vi "Que_Creat.vi"(8 "error in (no error)":errorcluster caption="error in", 11 "QueueName":string) -> (0 "error out":errorcluster, 3 "QueueName out":string)   [LabVIEW 2016]
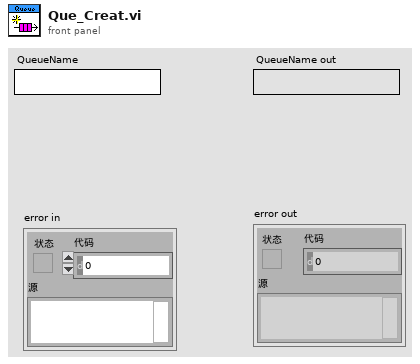
[diagram p1: front panel]
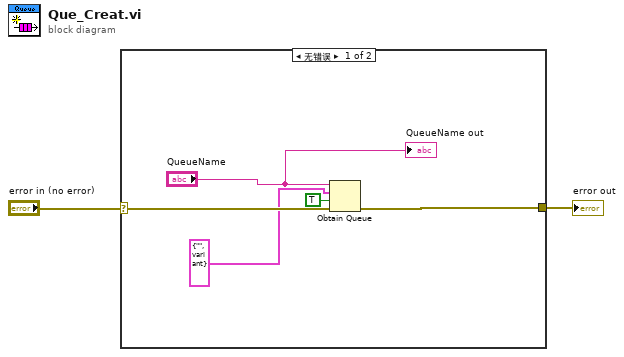
[diagram p0: block diagram]
diagram:
  n1 = case shown="无错误" "error in (no error)" {
    selector: "error in (no error)" -> [w7 w8]
    tunnel: [w5 w8] -> w1
    frame No Error {
      n2 = Obtain Queue(name (unnamed)="QueueName", element data type=cluster{string, "变体":variant} {"", "变体"=variant}, create if not found? (T)=TRUE ("如未找到是否创建？(T)"), error in (no error)=w7) -> (error out=w5:errorcluster)  [unwired: 1 in, 2 out]
      "QueueName out" <- "QueueName"
    }
    frame Error {
    }
  }
  "error out" <- w1
